vi "MC AO and DO Engine.vi"(0 "Unique Notifier Name":string="Not a Name", 11 "AO Channel":string[](array[string])) -> ()   [LabVIEW 2020]
uses:
  External Power Control Type Defs/External Power Notifier Type.ctl
  External Power Control Type Defs/External Power Actions.ctl
  <vilib>/ULx/Create Channel.llb/ULx Create Channel (DO-Digital Output).vi
  <vilib>/ULx/Write.llb/ULx Write (Digital Bool 1Line 1Point).vi
  <vilib>/ULx/Create Channel.llb/ULx Create Channel (AO-Voltage-Basic).vi
  <vilib>/ULx/Write.llb/ULx Write (Analog 1D DBL 1Chan 1Samp).vi
panel:
  in  "Power (%)":dbl
  in  "Quit":bool
  in  "Line On Off":bool
  # "Array Elements must be:\n\n1) AO Channel (e.g. Dev0/Ao0)\n2) DO Channel (e.g. Dev0/AuxPort/Do3)"
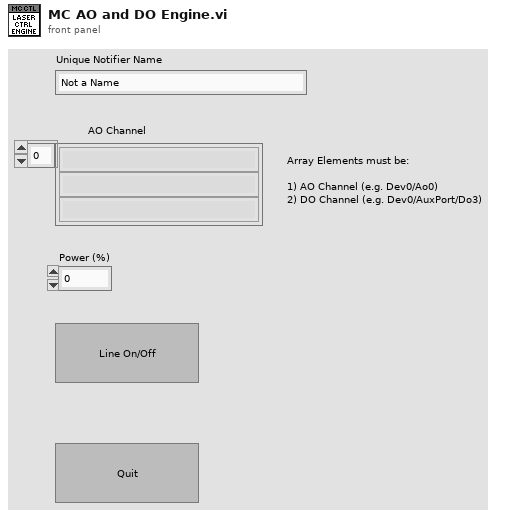
[diagram p1: front panel]
types:
  T1 = typedef "External Power Notifier Type.ctl" = cluster{"Actions":T2, "Wavelength":string, "Line On/Off":bool, "Power (%)":dbl, "Control Parameters":variant, "Cmd Done?":bool}
  T2 = typedef "External Power Actions.ctl" = enum16{"Line On/Off", "Set Power", "Set Ctrl Parameters", "Quit"}
  T3 = enum32{"Invalid", "Standard", "Closed", "Hidden", "Minimized", "Maximized"}
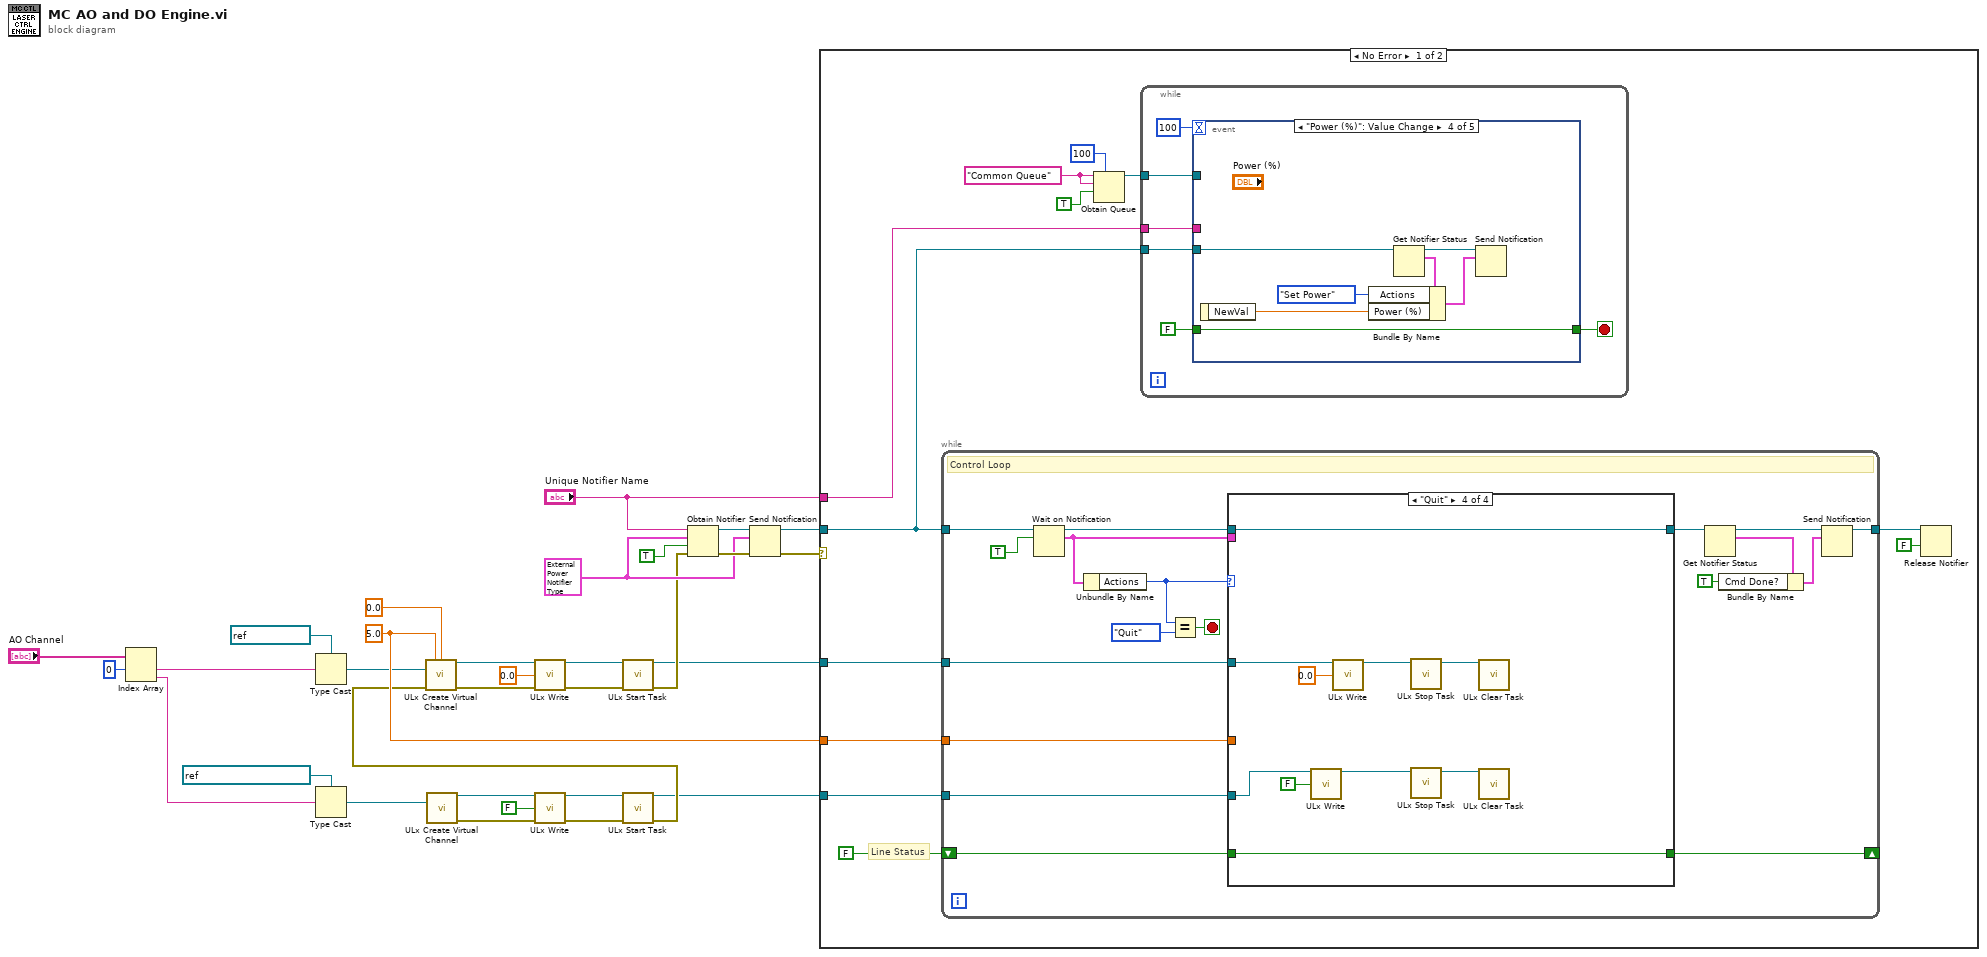
[diagram p0: block diagram]
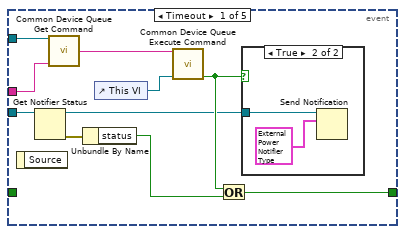
[diagram p2: hidden frame]
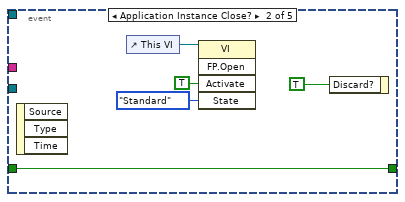
[diagram p4: hidden frame]
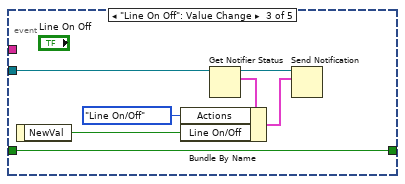
[diagram p5: hidden frame]
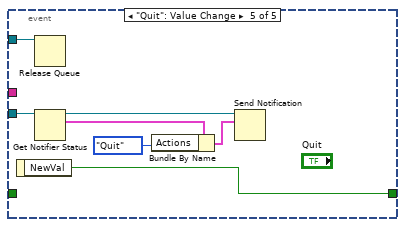
[diagram p6: hidden frame]
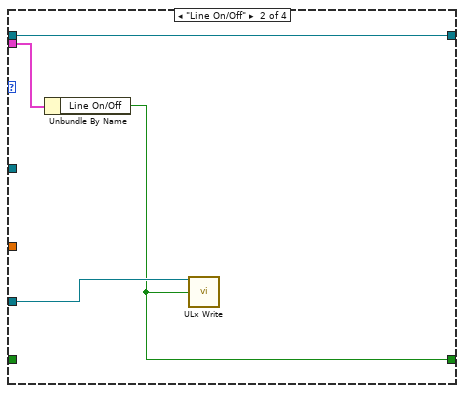
[diagram p8: hidden frame]
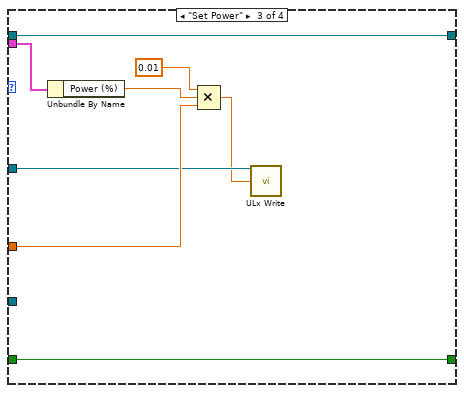
[diagram p9: hidden frame]
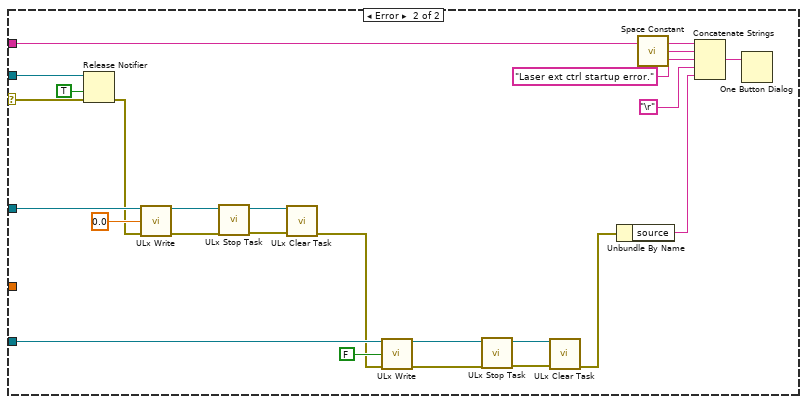
[diagram p10: hidden frame]
diagram:
  w22 = 5.0 ("maximum value")
  w27 = T1 {"Actions"=enum."Set Power", "Wavelength"="", "Line On/Off"=FALSE, "Power (%)"=0.0, "Control Parameters"=variant, "Cmd Done?"=FALSE} ("External Ctrl")
  n1 = Index Array(array="AO Channel", index #1=0 ("index")) -> (element #1=w20:string, element #2=w17:string)  [unwired: 1 in]
  n2 = Type Cast(type=refnum<k21> "Dev0/Ao0" ("physical channels"), x=w20) -> (*(type *) &x=w15:refnum<k21>)
  n3 = Type Cast(type=refnum<k21> "Dev0/AuxPort/Do0" ("lines"), x=w17) -> (*(type *) &x=w16:refnum<k21>)
  n4 = call-poly <vilib>:"ULx Create Virtual Channel.vi"("lines"=w16) -> ("task out"=w7:refnum<k24>, "error out"=w5:errorcluster)  [unwired: 13 in]
  n5 = call-poly <vilib>:"ULx Write.vi"("task in"=w7, "data"=FALSE, "error in"=w5) -> ("task out"=w4:refnum<k24>, "error out"=w3:errorcluster)  [unwired: 10 in, 1 out]
  n6 = call <vilib>:"ULx Start Task.vi"("task in"=w4, "error in"=w3) -> ("task out"=w1:refnum<k24>, "error out"=w2:errorcluster)  [unwired: 12 in]
  n7 = call-poly <vilib>:"ULx Create Virtual Channel.vi"("maximum value"=w22, "minimum value"=0.0, "physical channels"=w15, "error in"=w2) -> ("task out"=w14:refnum<k24>, "error out"=w13:errorcluster)  [unwired: 10 in]
  n8 = call-poly <vilib>:"ULx Write.vi"("task in"=w14, "data"=0.0, "error in"=w13) -> ("task out"=w11:refnum<k24>, "error out"=w10:errorcluster)  [unwired: 10 in, 1 out]
  n9 = call <vilib>:"ULx Start Task.vi"("task in"=w11, "error in"=w10) -> ("task out"=w8:refnum<k24>, "error out"=w9:errorcluster)  [unwired: 12 in]
  n10 = Obtain Notifier(name (unnamed)="Unique Notifier Name", notification data type=w27, create if not found? (T)=TRUE, error in (no error)=w9) -> (notifier out=w30:refnum<notifier>, error out=w29:errorcluster)  [unwired: 1 out]
  n11 = Send Notification(notification=w27, notifier=w30, error in (no error)=w29) -> (notifier out=w28:refnum<notifier>, error out=w26:errorcluster)
  n12 = case shown="No Error" w26 {
    selector: w26 -> [_ w151]
    tunnel: w8 -> [w43 w138]
    tunnel: w28 -> [w41 w152]
    tunnel: "Unique Notifier Name" -> [w40 w150]
    tunnel: w22 -> [w34 _]
    tunnel: w1 -> [w32 w137]
    frame No Error {
      w39 = "Common Queue" ("Unique Notifier Name")
      # "Line Status"
      n13 = while {
        tunnel: w41 -> [w97]
        tunnel: w43 -> [w103]
        tunnel: [w98] -> w33
        shift-right: [w90] -> _
        shift-left: FALSE -> [w91]
        tunnel: w34 -> [w89]
        tunnel: w32 -> [w88]
        stop <- w104 stop-if-true
        # "Control Loop"
        n14 = Wait on Notification(notifier=w97, ignore previous (F)=TRUE) -> (notifier out=w96:refnum<notifier>, notification=w95:T1)  [unwired: 2 in, 2 out]
        n15 = Unbundle By Name(w95) -> ("Actions"=w94:T2)
        n16 = Equal?(x=w94, y=External_Power_Actions."Quit") -> (x = y?=w104:bool)
        n17 = case shown="\"Quit\"" w94 {
          tunnel: w96 -> [w107 w111 w119 w129]
          tunnel: w103 -> [_ _ w113 w127]
          tunnel: [w107 w111 w119 w129] -> w101
          tunnel: w95 -> [_ w110 w118 _]
          tunnel: w91 -> [w106 _ w115 w128]
          tunnel: [w106 w108 w115 w128] -> w90
          tunnel: w89 -> [_ _ w114 _]
          tunnel: w88 -> [_ w109 _ w126]
          frame Default {
          }
          frame "Line On/Off" {
            n18 = Unbundle By Name(w110) -> ("Line On/Off"=w108:bool)
            n19 = call-poly <vilib>:"ULx Write.vi"("task in"=w109, "data"=w108) -> ()  [unwired: 11 in, 3 out]
          }
          frame "Set Power" {
            n20 = Unbundle By Name(w118) -> ("Power (%)"=w117:dbl)
            n21 = Compound Arithmetic op=MULTIPLY(0.01 ("value"), w117, w114) -> (w112:dbl)
            n22 = call-poly <vilib>:"ULx Write.vi"("task in"=w113, "data"=w112) -> ()  [unwired: 11 in, 3 out]
          }
          frame "Quit" {
            n23 = call-poly <vilib>:"ULx Write.vi"("task in"=w126, "data"=FALSE) -> ("task out"=w122:refnum<k24>)  [unwired: 11 in, 2 out]
            n24 = call-poly <vilib>:"ULx Write.vi"("task in"=w127, "data"=0.0) -> ("task out"=w123:refnum<k24>)  [unwired: 11 in, 2 out]
            n25 = call <vilib>:"ULx Stop Task.vi"("task in"=w123) -> ("task out"=w121:refnum<k24>)  [unwired: 9 in, 1 out]
            n26 = call <vilib>:"ULx Stop Task.vi"("task in"=w122) -> ("task out"=w120:refnum<k24>)  [unwired: 9 in, 1 out]
            n27 = call <vilib>:"ULx Clear Task.vi"("task in"=w121) -> ()  [unwired: 14 in, 1 out]
            n28 = call <vilib>:"ULx Clear Task.vi"("task in"=w120) -> ()  [unwired: 14 in, 1 out]
          }
        }
        n29 = Get Notifier Status(notifier=w101) -> (notifier out=w99:refnum<notifier>, current notification=w102:T1)  [unwired: 1 in, 3 out]
        n30 = Bundle By Name(cluster=w102, "Cmd Done?"=TRUE ("Received?")) -> (w92:T1)
        n31 = Send Notification(notification=w92, notifier=w99) -> (notifier out=w98:refnum<notifier>)  [unwired: 1 in, 1 out]
      }
      n32 = Obtain Queue(max queue size (-1, unlimited)=100, name (unnamed)=w39, element data type=w39, create if not found? (T)=TRUE) -> (queue out=w36:refnum<queue>)  [unwired: 1 in, 2 out]
      n33 = while {
        tunnel: w36 -> [w49]
        tunnel: w41 -> [w46]
        tunnel: w40 -> [w44]
        stop <- w45 stop-if-true
        n34 = event shown="[3] \"Power (%)\": Value Change" {
          selector: _ -> [_ _ _ _ _]
          dyn-events: _ -> [_ _ _ _ _]
          timeout: 100 -> [_ _ _ _ _]
          tunnel: w49 -> [w57 _ _ _ w82]
          tunnel: FALSE -> [_ w66 w69 w76 _]
          tunnel: w46 -> [w59 _ w73 w80 w83]
          tunnel: [w52 w66 w69 w76 w87] -> w45
          tunnel: w44 -> [w56 _ _ _ _]
          event Timeout {
            n35 = event-data() -> ()  [unwired: 1 in, 1 out]
            n36 = Get Notifier Status(notifier=w59) -> (notifier out=w50:refnum<notifier>, error out=w58:errorcluster)  [unwired: 1 in, 3 out]
            n37 = call "Common Device Queue Get Command.vi"("Common Queue"=w57, "Notifier Name"=w56) -> ("Command"=w55:string)  [unwired: 12 in, 1 out]
            n38 = Unbundle By Name(w58) -> ("status"=w53:bool)
            n39 = control-ref of="This VI"() -> (w54:refnum<vi>)
            n40 = call "Common Device Queue Execute Command.vi"("Common Command"=w55, "VI Refnum"=w54) -> ("Quit?"=w51:bool)  [unwired: 12 in, 1 out]
            n41 = Or(x=w51, y=w53) -> (x .or. y?=w52:bool)
            n42 = case shown="True" w51 {
              tunnel: w50 -> [_ w61]
              frame False {
              }
              frame True {
                n43 = Send Notification(notification=T1 {"Actions"=enum."Quit", "Wavelength"="", "Line On/Off"=FALSE, "Power (%)"=0.0, "Control Parameters"=variant, "Cmd Done?"=FALSE} ("External Ctrl"), notifier=w61) -> ()  [unwired: 1 in, 2 out]
              }
            }
          }
          event Application Instance Close? {
            n44 = event-data() -> ()  [unwired: 1 in, 3 out]
            n45 = control-ref of="This VI"() -> (w63:refnum<vi>)
            n46 = invoke class="VI" method="FP.Open"(reference=w63, "Activate"=TRUE ("Activate?"), "State"=T3."Standard") -> ()  [unwired: 2 in, 5 out]
            n47 = event-data("Discard?"=TRUE) -> ()  [unwired: 1 in, 1 out]
          }
          event "Line On Off": Value Change {
            n48 = event-data() -> ("NewVal"=w68:bool)  [unwired: 1 in]
            n49 = Get Notifier Status(notifier=w73) -> (notifier out=w72:refnum<notifier>, current notification=w71:T1)  [unwired: 1 in, 3 out]
            n50 = Bundle By Name(cluster=w71, "Actions"=External_Power_Actions."Line On/Off", "Line On/Off"=w68) -> (w70:T1)
            n51 = Send Notification(notification=w70, notifier=w72) -> ()  [unwired: 1 in, 2 out]
          }
          event "Power (%)": Value Change {
            n52 = event-data() -> ("NewVal"=w75:dbl)  [unwired: 1 in]
            n53 = Get Notifier Status(notifier=w80) -> (notifier out=w79:refnum<notifier>, current notification=w78:T1)  [unwired: 1 in, 3 out]
            n54 = Bundle By Name(cluster=w78, "Actions"=External_Power_Actions."Set Power", "Power (%)"=w75) -> (w77:T1)
            n55 = Send Notification(notification=w77, notifier=w79) -> ()  [unwired: 1 in, 2 out]
          }
          event "Quit": Value Change {
            n56 = event-data() -> ("NewVal"=w87:bool)  [unwired: 1 in]
            n57 = Release Queue(queue=w82) -> ()  [unwired: 2 in, 3 out]
            n58 = Get Notifier Status(notifier=w83) -> (notifier out=w86:refnum<notifier>, current notification=w85:T1)  [unwired: 1 in, 3 out]
            n59 = Bundle By Name(cluster=w85, "Actions"=External_Power_Actions."Quit") -> (w84:T1)
            n60 = Send Notification(notification=w84, notifier=w86) -> ()  [unwired: 1 in, 2 out]
          }
        }
      }
      n61 = Release Notifier(notifier=w33, force destroy? (F)=FALSE) -> ()  [unwired: 1 in, 3 out]
    }
    frame Error {
      n62 = Release Notifier(notifier=w152, force destroy? (F)=TRUE, error in (no error)=w151) -> (error out=w136:errorcluster)  [unwired: 2 out]
      n63 = call-poly <vilib>:"ULx Write.vi"("task in"=w138, "data"=0.0, "error in"=w136) -> ("task out"=w142:refnum<k24>, "error out"=w135:errorcluster)  [unwired: 10 in, 1 out]
      n64 = call <vilib>:"ULx Stop Task.vi"("error in"=w135, "task in"=w142) -> ("error out"=w134:errorcluster, "task out"=w140:refnum<k24>)  [unwired: 8 in]
      n65 = call <vilib>:"ULx Clear Task.vi"("task in"=w140, "error in"=w134) -> ("error out"=w133:errorcluster)  [unwired: 13 in]
      n66 = call-poly <vilib>:"ULx Write.vi"("task in"=w137, "data"=FALSE, "error in"=w133) -> ("task out"=w141:refnum<k24>, "error out"=w132:errorcluster)  [unwired: 10 in, 1 out]
      n67 = call <vilib>:"ULx Stop Task.vi"("error in"=w132, "task in"=w141) -> ("error out"=w131:errorcluster, "task out"=w139:refnum<k24>)  [unwired: 8 in]
      n68 = call <vilib>:"ULx Clear Task.vi"("task in"=w139, "error in"=w131) -> ("error out"=w130:errorcluster)  [unwired: 13 in]
      n69 = Unbundle By Name(w130) -> ("source"=w145:string)
      n70 = call <vilib>:"Space Constant.vi"() -> ("String"=w148:string)
      n71 = Concatenate Strings(w150, w148, "Laser ext ctrl startup error." ("string"), "\r", w145) -> (w149:string)
      n72 = One Button Dialog(message=w149) -> ()  [unwired: 1 in, 1 out]
    }
  }
